vi "Remove All Waveforms.vi"(8 "Error in":errorcluster, 11 "Custom Device ref":T1 format="%.0x") -> (0 "Error out":errorcluster, 3 "Custom Device ref out":T1 format="%.0x")   [LabVIEW 2015, in "Waveform-Processing-Custom-Device System Explorer.lvlib"]
uses:
  Waveform-Processing-Custom-Device System Explorer.lvlib
  <vilib>/NI Veristand/Custom Device API/Custom Device Item Ref.ctl
  <vilib>/NI VeriStand/Custom Device API/Custom Device API.lvlib
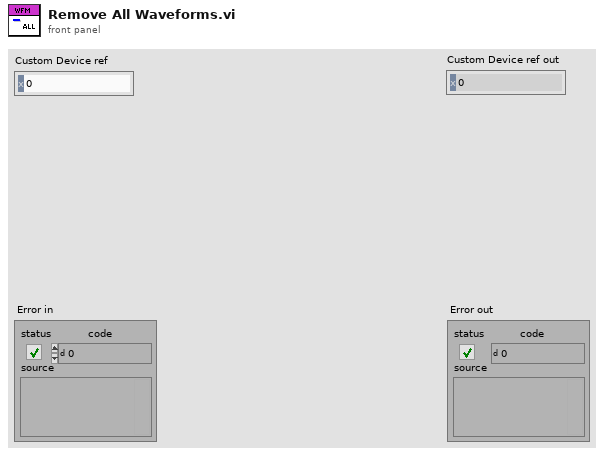
[diagram p1: front panel]
types:
  T1 = typedef "Custom Device API.lvlib/Custom Device Item Ref.ctl" = u64
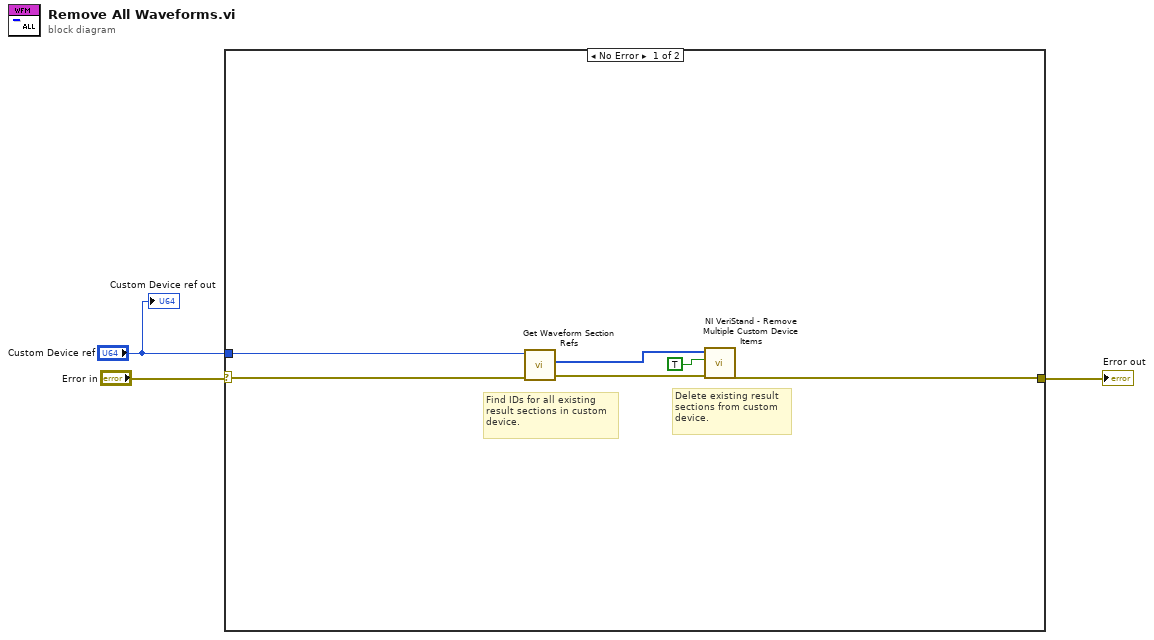
[diagram p0: block diagram]
diagram:
  n1 = case shown="No Error" "Error in" {
    selector: "Error in" -> [w9 w10]
    tunnel: "Custom Device ref" -> [w8 _]
    tunnel: [w5 w10] -> w2
    frame No Error {
      # "Delete existing result\nsections from custom\ndevice."
      # "Find IDs for all existing\nresult sections in custom\ndevice."
      n2 = call "Get Waveform Section Refs.vi"("Error in"=w9, "Device Ref in"=w8) -> ("Error out"=w7:errorcluster, "Result Section Refs"=w6:T1[])  [unwired: 7 in, 1 out]
      n3 = call <vilib>:"NI VeriStand - Remove Multiple Custom Device Items.vi"("error in (no error)"=w7, "Force Delete (F)"=TRUE, "Item Refs in"=w6) -> ("error out"=w5:errorcluster)  [unwired: 7 in, 1 out]
    }
    frame Error {
    }
  }
  "Error out" <- w2
  "Custom Device ref out" <- "Custom Device ref"
